vi "SetGainSpeed.vi"(1 "Gain":i32=1 min=1 max=10) -> (0 "Error":bool)   [LabVIEW 2014]
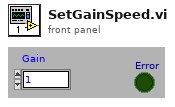
[diagram p1: front panel]
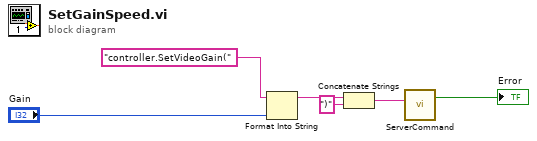
[diagram p0: block diagram]
diagram:
  n1 = Format Into String(initial string="controller.SetVideoGain(" ("Command"), "Gain") -> (resulting string=w3:string)  [unwired: 2 in, 1 out]
  n2 = Concatenate Strings(w3, ")" ("string")) -> (w1:string)
  n3 = call "ServerCommand.vi"("Command"=w1) -> ("Error"=→"Error":bool)  [unwired: 1 out]
